vi "build-diode-scan-pts - v2.vi"(4 "Bar In PD Angle":dbl=180.5 format="%#_13g", 5 "Test Start Delay (s)":dbl=60.0, 6 "Bar In Brewster Angle":dbl=45.0 format="%#_13g", 7 "queue in":T2(array[cluster]), 8 "PD Y":cluster{"stop":dbl, "start":dbl, "step":dbl}, 9 "PD X":cluster{"stop":dbl, "start":dbl, "step":dbl}, 10 "Bar Y":cluster{"stop":dbl, "start":dbl, "step":dbl}, 11 "Bar X":cluster{"stop":dbl, "start":dbl, "step":dbl}) -> (3 "queue out":T2(array[cluster]))   [LabVIEW 2024]
panel:
  in  "next-state-cluster":T1={"next-state"="", "mode-select"=enum."IR", "bypass-confirm"=FALSE, "PDX"=300.0, "PDY"=150.0, "BarX"=300.0, "BarY"=150.0, "BMA"=45.0, "PDA"=85.0, "bar-note"=FALSE}
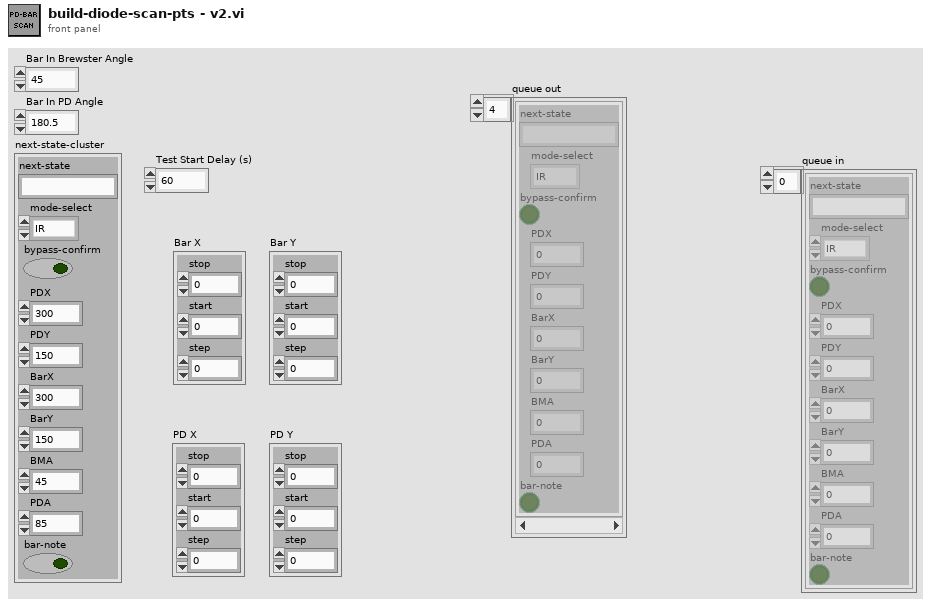
[diagram p1: front panel]
types:
  T1 = cluster{"next-state":string, "mode-select":enum32{"IR", "Pure", "Bulk", "Bar Out", "stored-loc", "custom"}, "bypass-confirm":bool, "PDX":dbl, "PDY":dbl, "BarX":dbl, "BarY":dbl, "BMA":dbl, "PDA":dbl, "bar-note":bool}
  T2 = cluster{"next-state":string, "mode-select":enum32{"IR", "Pure", "Bulk", "Bar Out", "stored-loc", "custom"}, "bypass-confirm":bool, "PDX":dbl, "PDY":dbl, "BarX":dbl, "BarY":dbl, "BMA":dbl, "PDA":dbl, "bar-note":bool}[]
  T3 = enum32{"IR", "Pure", "Bulk", "Bar Out", "stored-loc", "custom"}
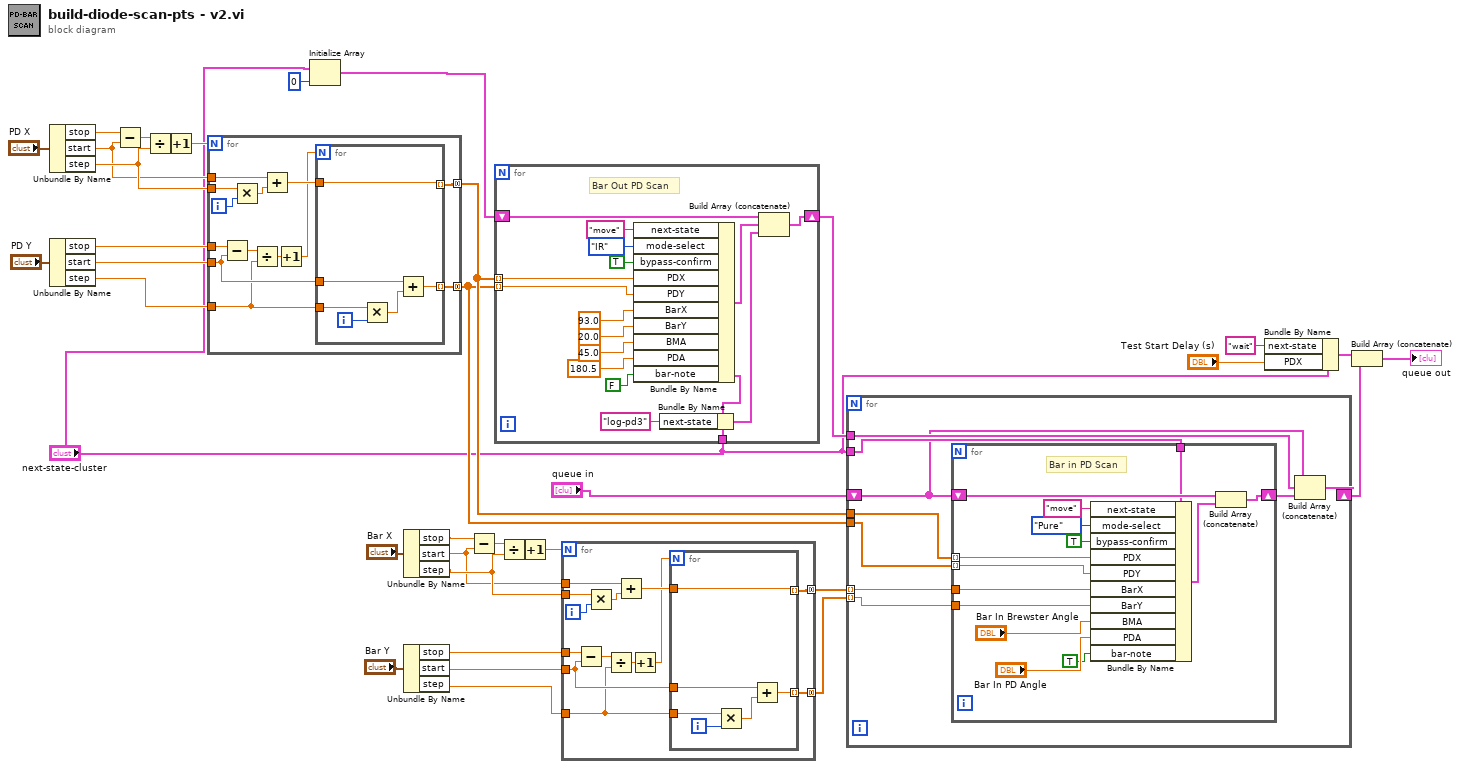
[diagram p0: block diagram]
diagram:
  n1 = Unbundle By Name("PD X") -> ("stop"=w16:dbl, "start"=w17:dbl, "step"=w18:dbl)
  n2 = Unbundle By Name("PD Y") -> ("stop"=w19:dbl, "start"=w20:dbl, "step"=w21:dbl)
  n3 = Subtract(x=w16, y=w17) -> (x-y=w10:dbl)
  n4 = Divide(x=w10, y=w18) -> (x/y=w11:dbl)
  n5 = Increment(x=w11) -> (x+1=w12:dbl)
  n6 = for {
    N: w12 -> [_]
    tunnel: w17 -> [w48]
    tunnel: [w45] -> w7 mode=concatenating
    tunnel: [w44] -> w6 mode=concatenating
    tunnel: w18 -> [w40]
    tunnel: w19 -> [w39]
    tunnel: w20 -> [w38]
    tunnel: w21 -> [w37]
    i -> [w49]
    n7 = Subtract(x=w39, y=w38) -> (x-y=w43:dbl)
    n8 = Multiply(x=w40, y=w49) -> (x*y=w47:dbl)
    n9 = Divide(x=w43, y=w37) -> (x/y=w42:dbl)
    n10 = Add(x=w48, y=w47) -> (x+y=w46:dbl)
    n11 = Increment(x=w42) -> (x+1=w41:dbl)
    n12 = for {
      N: w41 -> [_]
      tunnel: w46 -> [w55]
      tunnel: [w55] -> w45 mode=indexing
      tunnel: [w52] -> w44 mode=indexing
      tunnel: w38 -> [w51]
      tunnel: w37 -> [w50]
      i -> [w53]
      n13 = Multiply(x=w50, y=w53) -> (x*y=w54:dbl)
      n14 = Add(x=w51, y=w54) -> (x+y=w52:dbl)
    }
  }
  n15 = Initialize Array("next-state-cluster", 0 ("dimension size")) -> (w4:T2)
  n16 = Unbundle By Name("Bar X") -> ("stop"=w22:dbl, "start"=w23:dbl, "step"=w24:dbl)
  n17 = Unbundle By Name("Bar Y") -> ("stop"=w25:dbl, "start"=w26:dbl, "step"=w27:dbl)
  n18 = Subtract(x=w22, y=w23) -> (x-y=w15:dbl)
  n19 = for {
    tunnel: w7 -> [w71] mode=indexing
    tunnel: w6 -> [w70] mode=indexing
    shift-right: [w63] -> w9
    shift-left: w4 -> [w65]
    tunnel: "next-state-cluster" -> [w57]
    # "Bar Out PD Scan"
    n20 = Bundle By Name(cluster=w57, "next-state"="move", "mode-select"=T3."IR", "bypass-confirm"=TRUE, "PDX"=w71, "PDY"=w70, "BarX"=93.0, "BarY"=20.0, "BMA"=45.0, "PDA"=180.5, "bar-note"=FALSE) -> (w64:T1)
    n21 = Bundle By Name(cluster=w57, "next-state"="log-pd3") -> (w58:T1)
    n22 = Build Array (concatenate)(w65, w64, w58) -> (w63:T2)
  }
  n23 = Divide(x=w15, y=w24) -> (x/y=w14:dbl)
  n24 = Increment(x=w14) -> (x+1=w13:dbl)
  n25 = for {
    N: w13 -> [_]
    tunnel: w23 -> [w83]
    tunnel: [w80] -> w33 mode=concatenating
    tunnel: [w79] -> w34 mode=concatenating
    tunnel: w24 -> [w75]
    tunnel: w25 -> [w74]
    tunnel: w26 -> [w73]
    tunnel: w27 -> [w72]
    i -> [w84]
    n26 = Subtract(x=w74, y=w73) -> (x-y=w78:dbl)
    n27 = Multiply(x=w75, y=w84) -> (x*y=w82:dbl)
    n28 = Divide(x=w78, y=w72) -> (x/y=w77:dbl)
    n29 = Add(x=w83, y=w82) -> (x+y=w81:dbl)
    n30 = Increment(x=w77) -> (x+1=w76:dbl)
    n31 = for {
      N: w76 -> [_]
      tunnel: w81 -> [w90]
      tunnel: [w90] -> w80 mode=indexing
      tunnel: [w87] -> w79 mode=indexing
      tunnel: w73 -> [w86]
      tunnel: w72 -> [w85]
      i -> [w88]
      n32 = Multiply(x=w85, y=w88) -> (x*y=w89:dbl)
      n33 = Add(x=w86, y=w89) -> (x+y=w87:dbl)
    }
  }
  n34 = for {
    tunnel: w33 -> [w99] mode=indexing
    tunnel: w34 -> [w98] mode=indexing
    shift-right: [w96] -> w8
    shift-left: "queue in" -> [w91]
    tunnel: w9 -> [w95]
    tunnel: w7 -> [w94]
    tunnel: w6 -> [w93]
    tunnel: "next-state-cluster" -> [w92]
    n35 = for {
      tunnel: w94 -> [w113] mode=indexing
      tunnel: w93 -> [w112] mode=indexing
      shift-right: [w106] -> w97
      shift-left: w91 -> [w108]
      tunnel: w99 -> [w103]
      tunnel: w98 -> [w102]
      tunnel: w92 -> [w101]
      # "Bar in PD Scan"
      n36 = Bundle By Name(cluster=w101, "next-state"="move", "mode-select"=T3."Pure", "bypass-confirm"=TRUE, "PDX"=w113, "PDY"=w112, "BarX"=w103, "BarY"=w102, "BMA"="Bar In Brewster Angle", "PDA"="Bar In PD Angle", "bar-note"=TRUE) -> (w107:T1)
      n37 = Build Array (concatenate)(w108, w107) -> (w106:T2)
    }
    n38 = Build Array (concatenate)(w91, w95, w97) -> (w96:T2)
  }
  n39 = Bundle By Name(cluster="next-state-cluster", "next-state"="wait", "PDX"="Test Start Delay (s)") -> (w32:T1)
  n40 = Build Array (concatenate)(w32, w8) -> (→"queue out":T2)
